vi "Enter Leonardo Bootloader.vi"(8 "Error In":errorcluster, 11 "VISA resource name":refnum<visa-resource-name>) -> (0 "Error Out":errorcluster, 2 "Found?":bool, 3 "VISA resource name":refnum<visa-resource-name>)   [LabVIEW 2014, in "LMH-LINX.lvlib"]
uses:
  <vilib>/MakerHub/LINX/LMH-LINX.lvlib
  <vilib>/Instr/_visa.llb/VISA Configure Serial Port (Instr).vi
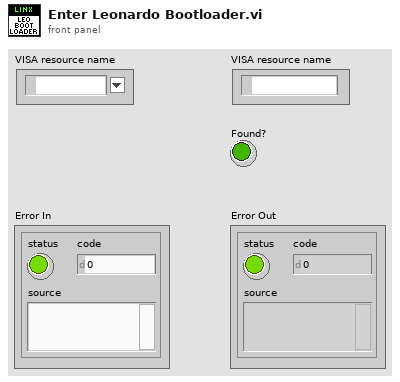
[diagram p1: front panel]
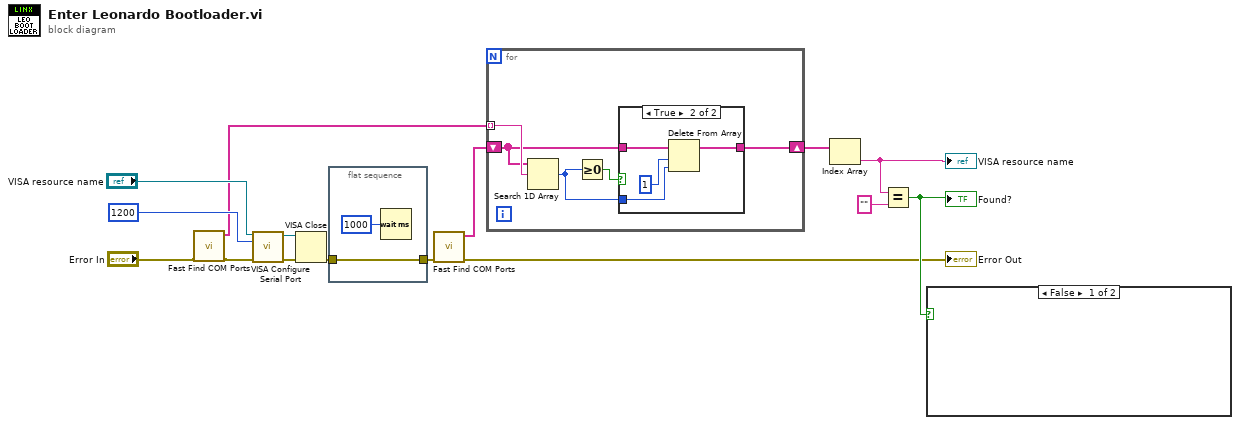
[diagram p0: block diagram]
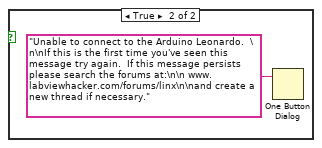
[diagram p3: hidden frame]
diagram:
  n1 = call <vilib>:"Fast Find COM Ports.vi"("Error In"="Error In") -> ("Error Out"=w6:errorcluster, "COM Ports"=w5:string[])  [unwired: 9 in]
  n2 = call-poly "VISA Configure Serial Port"("VISA resource name"="VISA resource name", "baud rate (9600)"=u32 1200, "error in (no error)"=w6) -> ("VISA resource name out"=w12:refnum<visa-resource-name>, "error out"=w13:errorcluster)  [unwired: 11 in]
  n3 = VISA Close(VISA resource name=w12, error in (no error)=w13) -> (error out=w1:errorcluster)
  n4 = flat-sequence {
    tunnel: [w17] -> w2
    tunnel: w1 -> [w17]
    frame #0 {
      n5 = Wait (ms)(milliseconds to wait=u32 1000) -> ()  [unwired: 1 out]
    }
  }
  n6 = call <vilib>:"Fast Find COM Ports.vi"("Error In"=w2) -> ("Error Out"=→"Error Out":errorcluster, "COM Ports"=w3:string[])  [unwired: 9 in]
  n7 = for {
    tunnel: w5 -> [w22] mode=indexing
    shift-right: [w21] -> w11
    shift-left: w3 -> [w20]
    n8 = Search 1D Array(1D array=w20, element=w22) -> (index of element=w19:i32)  [unwired: 1 in]
    n9 = Greater Or Equal To 0?(x=w19) -> (x >= 0?=w18:bool)
    n10 = case shown="True" w18 {
      tunnel: [w23 w27] -> w21
      tunnel: w20 -> [w23 w26]
      tunnel: w19 -> [_ w24]
      frame False {
      }
      frame True {
        n11 = Delete From Array(array=w26, length=1, index=w24) -> (array with subset deleted=w27:string[])  [unwired: 1 out]
      }
    }
  }
  n12 = Index Array(array=w11) -> (element=w8:string)  [unwired: 1 in]
  "VISA resource name" <- w8
  n13 = Equal?(x=w8, y="") -> (x = y?=w9:bool)
  "Found?" <- w9
  n14 = case shown="False" w9 {
    frame False {
    }
    frame True {
      n15 = One Button Dialog(message="Unable to connect to the Arduino Leonardo.  \n\nIf this is the first time you've seen this message try again.  If this message persists please search the forums at:\n\n www.labviewhacker.com/forums/linx\n\nand create a new thread if necessary.") -> ()  [unwired: 1 in, 1 out]
    }
  }
